vi "insert.vi"(8 "error in (no error)":errorcluster, 10 "data":dbl, 11 "node in":refnum<class "node.lvclass">) -> (0 "error out":errorcluster, 3 "node out":refnum<class "node.lvclass">)   [LabVIEW 2014, in "Linked List.lvlib" / "node.lvclass"]
uses:
  node.lvclass
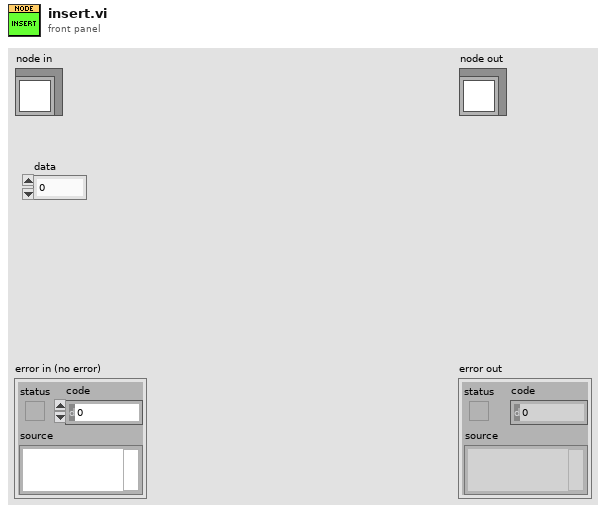
[diagram p1: front panel]
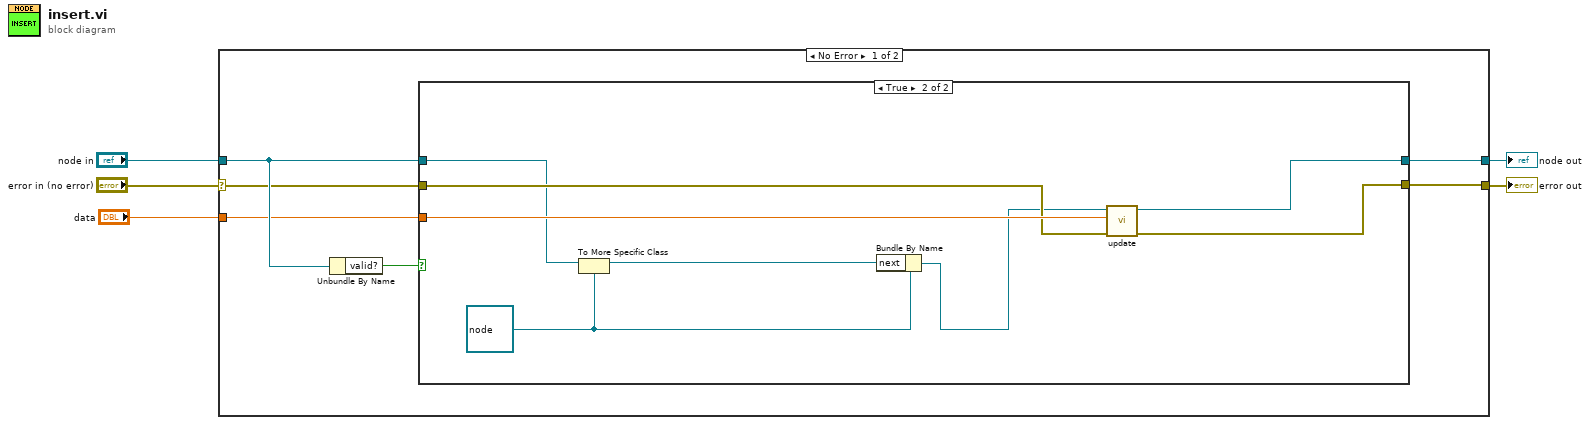
[diagram p0: block diagram]
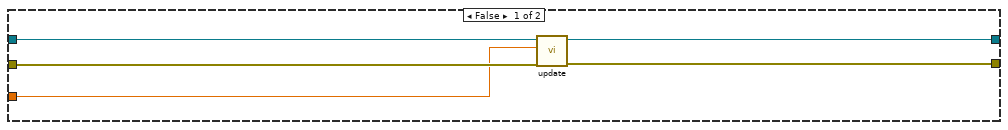
[diagram p2: hidden frame]
diagram:
  n1 = case shown="No Error" "error in (no error)" {
    selector: "error in (no error)" -> [w8 w26]
    tunnel: [w7 w26] -> w4
    tunnel: [w9 w25] -> w2
    tunnel: "node in" -> [w10 w25]
    tunnel: "data" -> [w6 _]
    frame No Error {
      n2 = Unbundle By Name(w10) -> ("valid?"=w11:bool)
      n3 = case shown="True" w11 {
        tunnel: w10 -> [w16 w19]
        tunnel: [w12 w17] -> w9
        tunnel: w8 -> [w15 w23]
        tunnel: [w14 w22] -> w7
        tunnel: w6 -> [w13 w24]
        frame False {
          n4 = call-dynamic "update.vi"("error in (no error)"=w15, "data"=w13, "node in"=w16) -> ("error out"=w14:errorcluster, "node out"=w12:refnum<class "node.lvclass">)  [unwired: 7 in]
        }
        frame True {
          w21 = refnum<class "node.lvclass"> refnum ("Linked List.lvlib:node")
          n5 = To More Specific Class(target class=w21, reference=w19) -> (specific class reference=w18:refnum<class "node.lvclass">)  [unwired: 1 in, 1 out]
          n6 = Bundle By Name(cluster=w21, "next"=w18) -> (w20:refnum<class "node.lvclass">)
          n7 = call-dynamic "update.vi"("error in (no error)"=w23, "data"=w24, "node in"=w20) -> ("error out"=w22:errorcluster, "node out"=w17:refnum<class "node.lvclass">)  [unwired: 7 in]
        }
      }
    }
    frame Error {
    }
  }
  "error out" <- w4
  "node out" <- w2
